vi "initialise.vi"(8 "error in (no error)":errorcluster, 11 "GenericImageProcessor in":refnum<class "GenericImageProcessor.lvclass">) -> (0 "error out":errorcluster, 3 "GenericImageProcessor out":refnum<class "GenericImageProcessor.lvclass">)   [LabVIEW 2010, in "GenericImageProcessor.lvclass"]
uses:
  GenericImageProcessor.lvclass
  common/classes/GenericComponent/GenericComponent/GenericComponent.lvclass
  GenericImageProcessor.lvclass/GenericImageProcessor.ctl
  common/classes/Image/Image/Image.lvclass
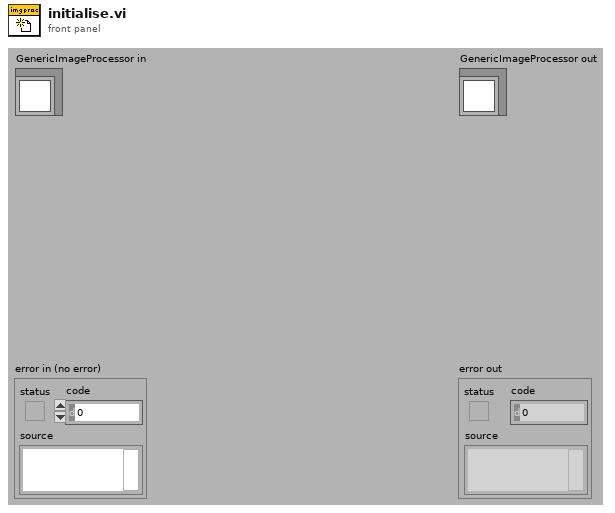
[diagram p1: front panel]
types:
  T1 = typedef "Image Type" = u32
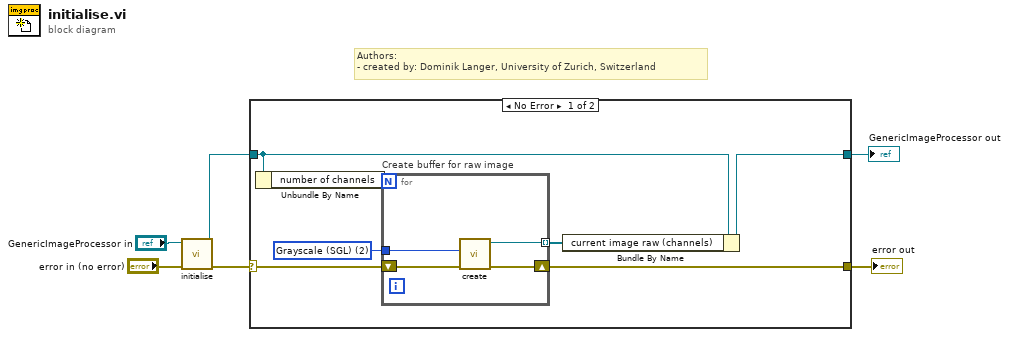
[diagram p0: block diagram]
diagram:
  # "Authors: \n- created by: Dominik Langer, University of Zurich, Switzerland"
  n1 = call-parent "initialise.vi"("error in (no error)"="error in (no error)", "GenericPlugin in"="GenericImageProcessor in") -> ("error out"=w3:errorcluster, "GenericPlugin out"=w1:refnum<class "GenericImageProcessor.lvclass">)  [unwired: 8 out]
  n2 = case shown="No Error" w3 {
    selector: w3 -> [w13 w19]
    tunnel: [w12 w19] -> w6
    tunnel: [w9 w18] -> w5
    tunnel: w1 -> [w10 w18]
    frame No Error {
      w7 = T1 2 items=["Grayscale (U8)", "Grayscale (I16)", "Grayscale (SGL)", "Complex (CSG)", "RGB (U32)", "HSL (U32)", "RGB (U64)", "Grayscale (U16)"] ("Image Type")
      n3 = Unbundle By Name(w10) -> ("number of channels"=w11:i32)
      n4 = for "Create buffer for raw image" {
        N: w11 -> [_]
        shift-right: [w16] -> w12
        shift-left: w13 -> [w17]
        tunnel: [w15] -> w8 mode=indexing
        tunnel: w7 -> [w14]
        n5 = call "create.vi"("error in (no error)"=w17, "Image Type"=w14) -> ("error out"=w16:errorcluster, "Image out"=w15:refnum<class "Image.lvclass">)  [unwired: 2 in, 6 out]
      }
      n6 = Bundle By Name(cluster=w10, "current image raw (channels)"=w8) -> (w9:refnum<class "GenericImageProcessor.lvclass">)
    }
    frame Error {
    }
  }
  "error out" <- w6
  "GenericImageProcessor out" <- w5
